vi "initialize.vi"(0 "HGF_SVSubscriber in":refnum<class "HGF_SVSubscriber.lvclass">, 3 "initializationData":variant, 5 "error in (no error)":errorcluster, 7 "binaryString":string, 8 "I8 Array":i8[](array[numeric]), 9 "prependSize? (T)":bool, 11 "byteOrder (0:big-endian, network order)":T1(ring)) -> (14 "HGF_SVSubscriber out":refnum<class "HGF_SVSubscriber.lvclass">, 17 "found?":bool, 19 "error out":errorcluster)   [LabVIEW 2012, in "HGF_SV.lvlib" / "HGF_SVSubscriber.lvclass"]
uses:
  HGF_SVSubscriber.lvclass
  DimLVEvent/LVDimInterface/LVDimInterface.dim service type.ctl
  HGF_BaseClasses/HGF_PVSubscriber/HGF_PVSubscriber.lvclass
  HGF_SVSubscriber.lvclass/HGF_SVSubscriber.ctl
  DimLVEvent/LVDimInterface/LVDimInterface.lvlib
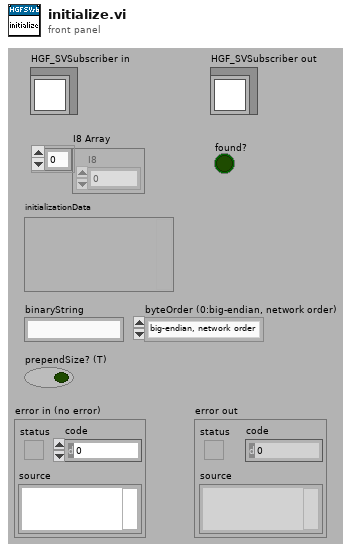
[diagram p1: front panel]
types:
  T1 = enum16{"big-endian, network order", "native, host order", "little-endian"}
  T2 = typedef "LVDimInterface.lvlib/LVDimInterface.dim service type.ctl" = u16
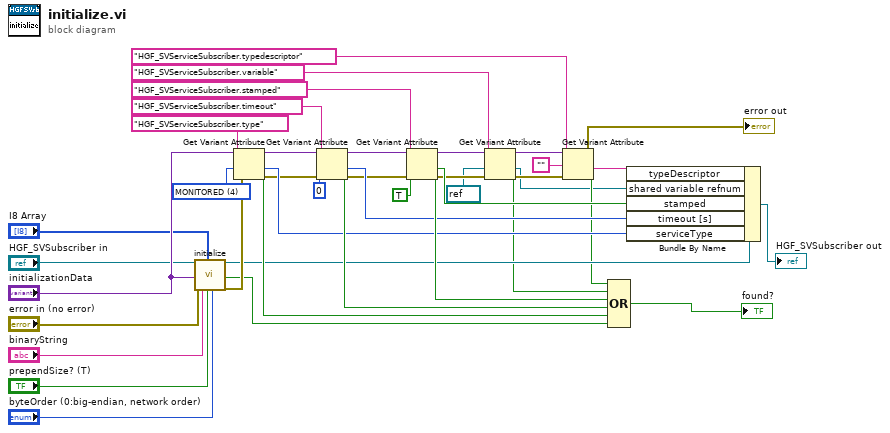
[diagram p0: block diagram]
diagram:
  w30 = T2 4 items=["ONCE_ONLY"=1, "TIMED"=2, "MONITORED"=4] ("typeOfDimService (monitored)")
  n1 = call-parent "initialize.vi"("HGV_PVBase"="HGF_SVSubscriber in", "initializationData"="initializationData", "error in (no error)"="error in (no error)", "binaryString"="binaryString", "I8 Array"="I8 Array", "prependSize? (T)"="prependSize? (T)", "byteOrder (0:big-endian, network order)"="byteOrder (0:big-endian, network order)") -> ("HGV_PVBase"=w16:refnum<class "HGF_SVSubscriber.lvclass">, "found?"=w36:bool, "error out"=w41:errorcluster)  [unwired: 10 out]
  n2 = Get Variant Attribute(Variant="initializationData", name="HGF_SVServiceSubscriber.type", default value (empty Variant)=w30, error in=w41) -> (duplicate Variant=w24:variant, found=w40:bool, value=w35:T2, error out=w25:errorcluster)
  n3 = Get Variant Attribute(Variant=w24, name="HGF_SVServiceSubscriber.timeout", default value (empty Variant)=0 ("timeout [0s]"), error in=w25) -> (duplicate Variant=w23:variant, found=w39:bool, value=w34:i32, error out=w26:errorcluster)
  n4 = Get Variant Attribute(Variant=w23, name="HGF_SVServiceSubscriber.stamped", default value (empty Variant)=TRUE ("stamped (T)"), error in=w26) -> (duplicate Variant=w12:variant, found=w38:bool, value=w33:bool, error out=w13:errorcluster)
  n5 = Get Variant Attribute(Variant=w12, name="HGF_SVServiceSubscriber.variable", default value (empty Variant)=refnum<k21> refnum ("shared variable refnum"), error in=w13) -> (duplicate Variant=w4:variant, found=w10:bool, value=w1:refnum<k21>, error out=w3:errorcluster)
  n6 = Get Variant Attribute(Variant=w4, name="HGF_SVServiceSubscriber.typedescriptor", default value (empty Variant)="", error in=w3) -> (found=w5:bool, value=w6:string, error out=→"error out":errorcluster)  [unwired: 1 out]
  n7 = Compound Arithmetic op=OR(w5, w10, w38, w39, w40, w36) -> (→"found?":bool)
  n8 = Bundle By Name(cluster=w16, "typeDescriptor"=w6, "shared variable refnum"=w1, "stamped"=w33, "timeout [s]"=w34, "serviceType"=w35) -> (→"HGF_SVSubscriber out":refnum<class "HGF_SVSubscriber.lvclass">)
